vi "23384_Davis_Poku_Amankwa_Amankwa.DavisPoku.MNE1201.6.6_348261_646291018.vi"() -> ()   [LabVIEW 2018]
panel:
  out "XY Graph":cluster{dbl[], dbl[]}(graph)
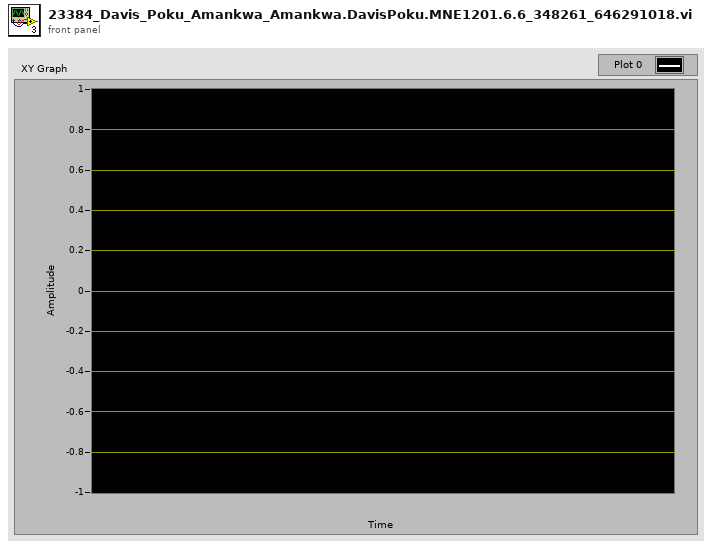
[diagram p1: front panel]
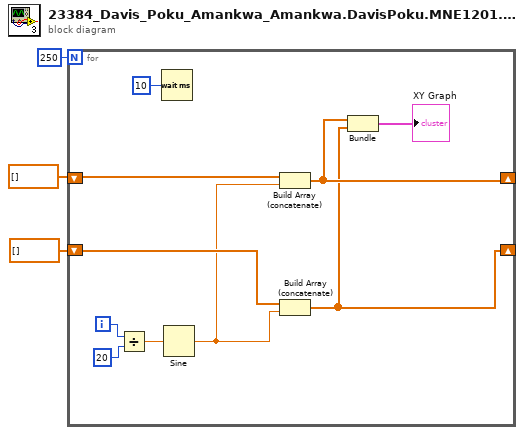
[diagram p0: block diagram]
diagram:
  n1 = for {
    N: 250 -> [_]
    shift-right: [w5] -> _
    shift-left: dbl[] [] -> [w7]
    shift-right: [w4] -> _
    shift-left: dbl[] [] -> [w9]
    i -> [w11]
    n2 = Divide(x=w11, y=20) -> (x/y=w10:dbl)
    n3 = Wait (ms)(milliseconds to wait=10) -> ()  [unwired: 1 out]
    n4 = Sine(x=w10) -> (sin(x)=w8:dbl)
    n5 = Build Array (concatenate)(w7, w8) -> (w5:dbl[])
    n6 = Build Array (concatenate)(w9, w8) -> (w4:dbl[])
    n7 = Bundle(w5, w4) -> (→"XY Graph":cluster{dbl[], dbl[]})  [unwired: 1 in]
  }
